vi "FipsAdjacent.vi"() -> (11 "Fips":i32[](array[numeric]))   [LabVIEW 2017] (continued)
MO\"\t29017\t\"Wayne County, MO\"\t29223\n\"Boone County, MO\"\t29019\t\"Audrain County, MO\"\t29007\n\"Boone County, MO\"\t29019\t\"Boone County, MO\"\t29019\n\"Boone County, MO\"\t29019\t\"Callaway County, MO\"\t29027\n\"Boone County, MO\"\t29019\t\"Cole County, MO\"\t29051\n\"Boone County, MO\"\t29019\t\"Cooper County, MO\"\t29053\n\"Boone County, MO\"\t29019\t\"Howard County, MO\"\t29089\n\"Boone County, MO\"\t29019\t\"Moniteau County, MO\"\t29135\n\"Boone County, MO\"\t29019\t\"Randolph County, MO\"\t29175\n\"Buchanan County, MO\"\t29021\t\"Atchison County, KS\"\t20005\n\"Buchanan County, MO\"\t29021\t\"Doniphan County, KS\"\t20043\n\"Buchanan County, MO\"\t29021\t\"Andrew County, MO\"\t29003\n\"Buchanan County, MO\"\t29021\t\"Buchanan County, MO\"\t29021\n\"Buchanan County, MO\"\t29021\t\"Clinton County, MO\"\t29049\n\"Buchanan County, MO\"\t29021\t\"DeKalb County, MO\"\t29063\n\"Buchanan County, MO\"\t29021\t\"Platte County, MO\"\t29165\n\"Butler County, MO\"\t29023\t\"Clay County, AR\"\t05021\n\"Butler County, MO\"\t29023\t\"Butler County, MO\"\t29023\n\"Butler County, MO\"\t29023\t\"Carter County, MO\"\t29035\n\"Butler County, MO\"\t29023\t\"Dunklin County, MO\"\t29069\n\"Butler County, MO\"\t29023\t\"Ripley County, MO\"\t29181\n\"Butler County, MO\"\t29023\t\"Stoddard County, MO\"\t29207\n\"Butler County, MO\"\t29023\t\"Wayne County, MO\"\t29223\n\"Caldwell County, MO\"\t29025\t\"Caldwell County, MO\"\t29025\n\"Caldwell County, MO\"\t29025\t\"Carroll County, MO\"\t29033\n\"Caldwell County, MO\"\t29025\t\"Clinton County, MO\"\t29049\n\"Caldwell County, MO\"\t29025\t\"Daviess County, MO\"\t29061\n\"Caldwell County, MO\"\t29025\t\"DeKalb County, MO\"\t29063\n\"Caldwell County, MO\"\t29025\t\"Livingston County, MO\"\t29117\n\"Caldwell County, MO\"\t29025\t\"Ray County, MO\"\t29177\n\"Callaway County, MO\"\t29027\t\"Audrain County, MO\"\t29007\n\"Callaway County, MO\"\t29027\t\"Boone County, MO\"\t29019\n\"Callaway County, MO\"\t29027\t\"Callaway County, MO\"\t29027\n\"Callaway County, MO\"\t29027\t\"Cole County, MO\"\t29051\n\"Callaway County, MO\"\t29027\t\"Montgomery County, MO\"\t29139\n\"Callaway County, MO\"\t29027\t\"Osage County, MO\"\t29151\n\"Camden County, MO\"\t29029\t\"Benton County, MO\"\t29015\n\"Camden County, MO\"\t29029\t\"Camden County, MO\"\t29029\n\"Camden County, MO\"\t29029\t\"Dallas County, MO\"\t29059\n\"Camden County, MO\"\t29029\t\"Hickory County, MO\"\t29085\n\"Camden County, MO\"\t29029\t\"Laclede County, MO\"\t29105\n\"Camden County, MO\"\t29029\t\"Miller County, MO\"\t29131\n\"Camden County, MO\"\t29029\t\"Morgan County, MO\"\t29141\n\"Camden County, MO\"\t29029\t\"Pulaski County, MO\"\t29169\n\"Cape Girardeau County, MO\"\t29031\t\"Alexander County, IL\"\t17003\n\"Cape Girardeau County, MO\"\t29031\t\"Union County, IL\"\t17181\n\"Cape Girardeau County, MO\"\t29031\t\"Bollinger County, MO\"\t29017\n\"Cape Girardeau County, MO\"\t29031\t\"Cape Girardeau County, MO\"\t29031\n\"Cape Girardeau County, MO\"\t29031\t\"Perry County, MO\"\t29157\n\"Cape Girardeau County, MO\"\t29031\t\"Scott County, MO\"\t29201\n\"Cape Girardeau County, MO\"\t29031\t\"Stoddard County, MO\"\t29207\n\"Carroll County, MO\"\t29033\t\"Caldwell County, MO\"\t29025\n\"Carroll County, MO\"\t29033\t\"Carroll County, MO\"\t29033\n\"Carroll County, MO\"\t29033\t\"Chariton County, MO\"\t29041\n\"Carroll County, MO\"\t29033\t\"Lafayette County, MO\"\t29107\n\"Carroll County, MO\"\t29033\t\"Livingston County, MO\"\t29117\n\"Carroll County, MO\"\t29033\t\"Ray County, MO\"\t29177\n\"Carroll County, MO\"\t29033\t\"Saline County, MO\"\t29195\n\"Carter County, MO\"\t29035\t\"Butler County, MO\"\t29023\n\"Carter County, MO\"\t29035\t\"Carter County, MO\"\t29035\n\"Carter County, MO\"\t29035\t\"Oregon County, MO\"\t29149\n\"Carter County, MO\"\t29035\t\"Reynolds County, MO\"\t29179\n\"Carter County, MO\"\t29035\t\"Ripley County, MO\"\t29181\n\"Carter County, MO\"\t29035\t\"Shannon County, MO\"\t29203\n\"Carter County, MO\"\t29035\t\"Wayne County, MO\"\t29223\n\"Cass County, MO\"\t29037\t\"Johnson County, KS\"\t20091\n\"Cass County, MO\"\t29037\t\"Miami County, KS\"\t20121\n\"Cass County, MO\"\t29037\t\"Bates County, MO\"\t29013\n\"Cass County, MO\"\t29037\t\"Cass County, MO\"\t29037\n\"Cass County, MO\"\t29037\t\"Henry County, MO\"\t29083\n\"Cass County, MO\"\t29037\t\"Jackson County, MO\"\t29095\n\"Cass County, MO\"\t29037\t\"Johnson County, MO\"\t29101\n\"Cedar County, MO\"\t29039\t\"Barton County, MO\"\t29011\n\"Cedar County, MO\"\t29039\t\"Cedar County, MO\"\t29039\n\"Cedar County, MO\"\t29039\t\"Dade County, MO\"\t29057\n\"Cedar County, MO\"\t29039\t\"Polk County, MO\"\t29167\n\"Cedar County, MO\"\t29039\t\"St. Clair County, MO\"\t29185\n\"Cedar County, MO\"\t29039\t\"Vernon County, MO\"\t29217\n\"Chariton County, MO\"\t29041\t\"Carroll County, MO\"\t29033\n\"Chariton County, MO\"\t29041\t\"Chariton County, MO\"\t29041\n\"Chariton County, MO\"\t29041\t\"Howard County, MO\"\t29089\n\"Chariton County, MO\"\t29041\t\"Linn County, MO\"\t29115\n\"Chariton County, MO\"\t29041\t\"Livingston County, MO\"\t29117\n\"Chariton County, MO\"\t29041\t\"Macon County, MO\"\t29121\n\"Chariton County, MO\"\t29041\t\"Randolph County, MO\"\t29175\n\"Chariton County, MO\"\t29041\t\"Saline County, MO\"\t29195\n\"Christian County, MO\"\t29043\t\"Christian County, MO\"\t29043\n\"Christian County, MO\"\t29043\t\"Douglas County, MO\"\t29067\n\"Christian County, MO\"\t29043\t\"Greene County, MO\"\t29077\n\"Christian County, MO\"\t29043\t\"Lawrence County, MO\"\t29109\n\"Christian County, MO\"\t29043\t\"Stone County, MO\"\t29209\n\"Christian County, MO\"\t29043\t\"Taney County, MO\"\t29213\n\"Christian County, MO\"\t29043\t\"Webster County, MO\"\t29225\n\"Clark County, MO\"\t29045\t\"Hancock County, IL\"\t17067\n\"Clark County, MO\"\t29045\t\"Lee County, IA\"\t19111\n\"Clark County, MO\"\t29045\t\"Van Buren County, IA\"\t19177\n\"Clark County, MO\"\t29045\t\"Clark County, MO\"\t29045\n\"Clark County, MO\"\t29045\t\"Knox County, MO\"\t29103\n\"Clark County, MO\"\t29045\t\"Lewis County, MO\"\t29111\n\"Clark County, MO\"\t29045\t\"Scotland County, MO\"\t29199\n\"Clay County, MO\"\t29047\t\"Wyandotte County, KS\"\t20209\n\"Clay County, MO\"\t29047\t\"Clay County, MO\"\t29047\n\"Clay County, MO\"\t29047\t\"Clinton County, MO\"\t29049\n\"Clay County, MO\"\t29047\t\"Jackson County, MO\"\t29095\n\"Clay County, MO\"\t29047\t\"Platte County, MO\"\t29165\n\"Clay County, MO\"\t29047\t\"Ray County, MO\"\t29177\n\"Clinton County, MO\"\t29049\t\"Buchanan County, MO\"\t29021\n\"Clinton County, MO\"\t29049\t\"Caldwell County, MO\"\t29025\n\"Clinton County, MO\"\t29049\t\"Clay County, MO\"\t29047\n\"Clinton County, MO\"\t29049\t\"Clinton County, MO\"\t29049\n\"Clinton County, MO\"\t29049\t\"DeKalb County, MO\"\t29063\n\"Clinton County, MO\"\t29049\t\"Platte County, MO\"\t29165\n\"Clinton County, MO\"\t29049\t\"Ray County, MO\"\t29177\n\"Cole County, MO\"\t29051\t\"Boone County, MO\"\t29019\n\"Cole County, MO\"\t29051\t\"Callaway County, MO\"\t29027\n\"Cole County, MO\"\t29051\t\"Cole County, MO\"\t29051\n\"Cole County, MO\"\t29051\t\"Miller County, MO\"\t29131\n\"Cole County, MO\"\t29051\t\"Moniteau County, MO\"\t29135\n\"Cole County, MO\"\t29051\t\"Osage County, MO\"\t29151\n\"Cooper County, MO\"\t29053\t\"Boone County, MO\"\t29019\n\"Cooper County, MO\"\t29053\t\"Cooper County, MO\"\t29053\n\"Cooper County, MO\"\t29053\t\"Howard County, MO\"\t29089\n\"Cooper County, MO\"\t29053\t\"Moniteau County, MO\"\t29135\n\"Cooper County, MO\"\t29053\t\"Morgan County, MO\"\t29141\n\"Cooper County, MO\"\t29053\t\"Pettis County, MO\"\t29159\n\"Cooper County, MO\"\t29053\t\"Saline County, MO\"\t29195\n\"Crawford County, MO\"\t29055\t\"Crawford County, MO\"\t29055\n\"Crawford County, MO\"\t29055\t\"Dent County, MO\"\t29065\n\"Crawford County, MO\"\t29055\t\"Franklin County, MO\"\t29071\n\"Crawford County, MO\"\t29055\t\"Gasconade County, MO\"\t29073\n\"Crawford County, MO\"\t29055\t\"Iron County, MO\"\t29093\n\"Crawford County, MO\"\t29055\t\"Phelps County, MO\"\t29161\n\"Crawford County, MO\"\t29055\t\"Washington County, MO\"\t29221\n\"Dade County, MO\"\t29057\t\"Barton County, MO\"\t29011\n\"Dade County, MO\"\t29057\t\"Cedar County, MO\"\t29039\n\"Dade County, MO\"\t29057\t\"Dade County, MO\"\t29057\n\"Dade County, MO\"\t29057\t\"Greene County, MO\"\t29077\n\"Dade County, MO\"\t29057\t\"Jasper County, MO\"\t29097\n\"Dade County, MO\"\t29057\t\"Lawrence County, MO\"\t29109\n\"Dade County, MO\"\t29057\t\"Polk County, MO\"\t29167\n\"Dallas County, MO\"\t29059\t\"Camden County, MO\"\t29029\n\"Dallas County, MO\"\t29059\t\"Dallas County, MO\"\t29059\n\"Dallas County, MO\"\t29059\t\"Greene County, MO\"\t29077\n\"Dallas County, MO\"\t29059\t\"Hickory County, MO\"\t29085\n\"Dallas County, MO\"\t29059\t\"Laclede County, MO\"\t29105\n\"Dallas County, MO\"\t29059\t\"Polk County, MO\"\t29167\n\"Dallas County, MO\"\t29059\t\"Webster County, MO\"\t29225\n\"Daviess County, MO\"\t29061\t\"Caldwell County, MO\"\t29025\n\"Daviess County, MO\"\t29061\t\"Daviess County, MO\"\t29061\n\"Daviess County, MO\"\t29061\t\"DeKalb County, MO\"\t29063\n\"Daviess County, MO\"\t29061\t\"Gentry County, MO\"\t29075\n\"Daviess County, MO\"\t29061\t\"Grundy County, MO\"\t29079\n\"Daviess County, MO\"\t29061\t\"Harrison County, MO\"\t29081\n\"Daviess County, MO\"\t29061\t\"Livingston County, MO\"\t29117\n\"DeKalb County, MO\"\t29063\t\"Andrew County, MO\"\t29003\n\"DeKalb County, MO\"\t29063\t\"Buchanan County, MO\"\t29021\n\"DeKalb County, MO\"\t29063\t\"Caldwell County, MO\"\t29025\n\"DeKalb County, MO\"\t29063\t\"Clinton County, MO\"\t29049\n\"DeKalb County, MO\"\t29063\t\"Daviess County, MO\"\t29061\n\"DeKalb County, MO\"\t29063\t\"DeKalb County, MO\"\t29063\n\"DeKalb County, MO\"\t29063\t\"Gentry County, MO\"\t29075\n\"Dent County, MO\"\t29065\t\"Crawford County, MO\"\t29055\n\"Dent County, MO\"\t29065\t\"Dent County, MO\"\t29065\n\"Dent County, MO\"\t29065\t\"Iron County, MO\"\t29093\n\"Dent County, MO\"\t29065\t\"Phelps County, MO\"\t29161\n\"Dent County, MO\"\t29065\t\"Reynolds County, MO\"\t29179\n\"Dent County, MO\"\t29065\t\"Shannon County, MO\"\t29203\n\"Dent County, MO\"\t29065\t\"Texas County, MO\"\t29215\n\"Douglas County, MO\"\t29067\t\"Christian County, MO\"\t29043\n\"Douglas County, MO\"\t29067\t\"Douglas County, MO\"\t29067\n\"Douglas County, MO\"\t29067\t\"Howell County, MO\"\t29091\n\"Douglas County, MO\"\t29067\t\"Ozark County, MO\"\t29153\n\"Douglas County, MO\"\t29067\t\"Taney County, MO\"\t29213\n\"Douglas County, MO\"\t29067\t\"Texas County, MO\"\t29215\n\"Douglas County, MO\"\t29067\t\"Webster County, MO\"\t29225\n\"Douglas County, MO\"\t29067\t\"Wright County, MO\"\t29229\n\"Dunklin County, MO\"\t29069\t\"Clay County, AR\"\t05021\n\"Dunklin County, MO\"\t29069\t\"Craighead County, AR\"\t05031\n\"Dunklin County, MO\"\t29069\t\"Greene County, AR\"\t05055\n\"Dunklin County, MO\"\t29069\t\"Mississippi County, AR\"\t05093\n\"Dunklin County, MO\"\t29069\t\"Butler County, MO\"\t29023\n\"Dunklin County, MO\"\t29069\t\"Dunklin County, MO\"\t29069\n\"Dunklin County, MO\"\t29069\t\"New Madrid County, MO\"\t29143\n\"Dunklin County, MO\"\t29069\t\"Pemiscot County, MO\"\t29155\n\"Dunklin County, MO\"\t29069\t\"Stoddard County, MO\"\t29207\n\"Franklin County, MO\"\t29071\t\"Crawford County, MO\"\t29055\n\"Franklin County, MO\"\t29071\t\"Franklin County, MO\"\t29071\n\"Franklin County, MO\"\t29071\t\"Gasconade County, MO\"\t29073\n\"Franklin County, MO\"\t29071\t\"Jefferson County, MO\"\t29099\n\"Franklin County, MO\"\t29071\t\"St. Charles County, MO\"\t29183\n\"Franklin County, MO\"\t29071\t\"St. Louis County, MO\"\t29189\n\"Franklin County, MO\"\t29071\t\"Warren County, MO\"\t29219\n\"Franklin County, MO\"\t29071\t\"Washington County, MO\"\t29221\n\"Gasconade County, MO\"\t29073\t\"Crawford County, MO\"\t29055\n\"Gasconade County, MO\"\t29073\t\"Franklin County, MO\"\t29071\n\"Gasconade County, MO\"\t29073\t\"Gasconade County, MO\"\t29073\n\"Gasconade County, MO\"\t29073\t\"Maries County, MO\"\t29125\n\"Gasconade County, MO\"\t29073\t\"Montgomery County, MO\"\t29139\n\"Gasconade County, MO\"\t29073\t\"Osage County, MO\"\t29151\n\"Gasconade County, MO\"\t29073\t\"Phelps County, MO\"\t29161\n\"Gasconade County, MO\"\t29073\t\"Warren County, MO\"\t29219\n\"Gentry County, MO\"\t29075\t\"Andrew County, MO\"\t29003\n\"Gentry County, MO\"\t29075\t\"Daviess County, MO\"\t29061\n\"Gentry County, MO\"\t29075\t\"DeKalb County, MO\"\t29063\n\"Gentry County, MO\"\t29075\t\"Gentry County, MO\"\t29075\n\"Gentry County, MO\"\t29075\t\"Harrison County, MO\"\t29081\n\"Gentry County, MO\"\t29075\t\"Nodaway County, MO\"\t29147\n\"Gentry County, MO\"\t29075\t\"Worth County, MO\"\t29227\n\"Greene County, MO\"\t29077\t\"Christian County, MO\"\t29043\n\"Greene County, MO\"\t29077\t\"Dade County, MO\"\t29057\n\"Greene County, MO\"\t29077\t\"Dallas County, MO\"\t29059\n\"Greene County, MO\"\t29077\t\"Greene County, MO\"\t29077\n\"Greene County, MO\"\t29077\t\"Lawrence County, MO\"\t29109\n\"Greene County, MO\"\t29077\t\"Polk County, MO\"\t29167\n\"Greene County, MO\"\t29077\t\"Webster County, MO\"\t29225\n\"Grundy County, MO\"\t29079\t\"Daviess County, MO\"\t29061\n\"Grundy County, MO\"\t29079\t\"Grundy County, MO\"\t29079\n\"Grundy County, MO\"\t29079\t\"Harrison County, MO\"\t29081\n\"Grundy County, MO\"\t29079\t\"Linn County, MO\"\t29115\n\"Grundy County, MO\"\t29079\t\"Livingston County, MO\"\t29117\n\"Grundy County, MO\"\t29079\t\"Mercer County, MO\"\t29129\n\"Grundy County, MO\"\t29079\t\"Sullivan County, MO\"\t29211\n\"Harrison County, MO\"\t29081\t\"Decatur County, IA\"\t19053\n\"Harrison County, MO\"\t29081\t\"Ringgold County, IA\"\t19159\n\"Harrison County, MO\"\t29081\t\"Daviess County, MO\"\t29061\n\"Harrison County, MO\"\t29081\t\"Gentry County, MO\"\t29075\n\"Harrison County, MO\"\t29081\t\"Grundy County, MO\"\t29079\n\"Harrison County, MO\"\t29081\t\"Harrison County, MO\"\t29081\n\"Harrison County, MO\"\t29081\t\"Mercer County, MO\"\t29129\n\"Harrison County, MO\"\t29081\t\"Worth County, MO\"\t29227\n\"Henry County, MO\"\t29083\t\"Bates County, MO\"\t29013\n\"Henry County, MO\"\t29083\t\"Benton County, MO\"\t29015\n\"Henry County, MO\"\t29083\t\"Cass County, MO\"\t29037\n\"Henry County, MO\"\t29083\t\"Henry County, MO\"\t29083\n\"Henry County, MO\"\t29083\t\"Johnson County, MO\"\t29101\n\"Henry County, MO\"\t29083\t\"Pettis County, MO\"\t29159\n\"Henry County, MO\"\t29083\t\"St. Clair County, MO\"\t29185\n\"Hickory County, MO\"\t29085\t\"Benton County, MO\"\t29015\n\"Hickory County, MO\"\t29085\t\"Camden County, MO\"\t29029\n\"Hickory County, MO\"\t29085\t\"Dallas County, MO\"\t29059\n\"Hickory County, MO\"\t29085\t\"Hickory County, MO\"\t29085\n\"Hickory County, MO\"\t29085\t\"Polk County, MO\"\t29167\n\"Hickory County, MO\"\t29085\t\"St. Clair County, MO\"\t29185\n\"Holt County, MO\"\t29087\t\"Doniphan County, KS\"\t20043\n\"Holt County, MO\"\t29087\t\"Andrew County, MO\"\t29003\n\"Holt County, MO\"\t29087\t\"Atchison County, MO\"\t29005\n\"Holt County, MO\"\t29087\t\"Holt County, MO\"\t29087\n\"Holt County, MO\"\t29087\t\"Nodaway County, MO\"\t29147\n\"Holt County, MO\"\t29087\t\"Nemaha County, NE\"\t31127\n\"Holt County, MO\"\t29087\t\"Richardson County, NE\"\t31147\n\"Howard County, MO\"\t29089\t\"Boone County, MO\"\t29019\n\"Howard County, MO\"\t29089\t\"Chariton County, MO\"\t29041\n\"Howard County, MO\"\t29089\t\"Cooper County, MO\"\t29053\n\"Howard County, MO\"\t29089\t\"Howard County, MO\"\t29089\n\"Howard County, MO\"\t29089\t\"Randolph County, MO\"\t29175\n\"Howard County, MO\"\t29089\t\"Saline County, MO\"\t29195\n\"Howell County, MO\"\t29091\t\"Fulton County, AR\"\t05049\n\"Howell County, MO\"\t29091\t\"Douglas County, MO\"\t29067\n\"Howell County, MO\"\t29091\t\"Howell County, MO\"\t29091\n\"Howell County, MO\"\t29091\t\"Oregon County, MO\"\t29149\n\"Howell County, MO\"\t29091\t\"Ozark County, MO\"\t29153\n\"Howell County, MO\"\t29091\t\"Shannon County, MO\"\t29203\n\"Howell County, MO\"\t29091\t\"Texas County, MO\"\t29215\n\"Iron County, MO\"\t29093\t\"Crawford County, MO\"\t29055\n\"Iron County, MO\"\t29093\t\"Dent County, MO\"\t29065\n\"Iron County, MO\"\t29093\t\"Iron County, MO\"\t29093\n\"Iron County, MO\"\t29093\t\"Madison County, MO\"\t29123\n\"Iron County, MO\"\t29093\t\"Reynolds County, MO\"\t29179\n\"Iron County, MO\"\t29093\t\"St. Francois County, MO\"\t29187\n\"Iron County, MO\"\t29093\t\"Washington County, MO\"\t29221\n\"Iron County, MO\"\t29093\t\"Wayne County, MO\"\t29223\n\"Jackson County, MO\"\t29095\t\"Johnson County, KS\"\t20091\n\"Jackson County, MO\"\t29095\t\"Wyandotte County, KS\"\t20209\n\"Jackson County, MO\"\t29095\t\"Cass County, MO\"\t29037\n\"Jackson County, MO\"\t29095\t\"Clay County, MO\"\t29047\n\"Jackson County, MO\"\t29095\t\"Jackson County, MO\"\t29095\n\"Jackson County, MO\"\t29095\t\"Johnson County, MO\"\t29101\n\"Jackson County, MO\"\t29095\t\"Lafayette County, MO\"\t29107\n\"Jackson County, MO\"\t29095\t\"Ray County, MO\"\t29177\n\"Jasper County, MO\"\t29097\t\"Cherokee County, KS\"\t20021\n\"Jasper County, MO\"\t29097\t\"Crawford County, KS\"\t20037\n\"Jasper County, MO\"\t29097\t\"Barton County, MO\"\t29011\n\"Jasper County, MO\"\t29097\t\"Dade County, MO\"\t29057\n\"Jasper County, MO\"\t29097\t\"Jasper County, MO\"\t29097\n\"Jasper County, MO\"\t29097\t\"Lawrence County, MO\"\t29109\n\"Jasper County, MO\"\t29097\t\"Newton County, MO\"\t29145\n\"Jefferson County, MO\"\t29099\t\"Monroe County, IL\"\t17133\n\"Jefferson County, MO\"\t29099\t\"Franklin County, MO\"\t29071\n\"Jefferson County, MO\"\t29099\t\"Jefferson County, MO\"\t29099\n\"Jefferson County, MO\"\t29099\t\"Ste. Genevieve County, MO\"\t29186\n\"Jefferson County, MO\"\t29099\t\"St. Francois County, MO\"\t29187\n\"Jefferson County, MO\"\t29099\t\"St. Louis County, MO\"\t29189\n\"Jefferson County, MO\"\t29099\t\"Washington County, MO\"\t29221\n\"Johnson County, MO\"\t29101\t\"Cass County, MO\"\t29037\n\"Johnson County, MO\"\t29101\t\"Henry County, MO\"\t29083\n\"Johnson County, MO\"\t29101\t\"Jackson County, MO\"\t29095\n\"Johnson County, MO\"\t29101\t\"Johnson County, MO\"\t29101\n\"Johnson County, MO\"\t29101\t\"Lafayette County, MO\"\t29107\n\"Johnson County, MO\"\t29101\t\"Pettis County, MO\"\t29159\n\"Knox County, MO\"\t29103\t\"Adair County, MO\"\t29001\n\"Knox County, MO\"\t29103\t\"Clark County, MO\"\t29045\n\"Knox County, MO\"\t29103\t\"Knox County, MO\"\t29103\n\"Knox County, MO\"\t29103\t\"Lewis County, MO\"\t29111\n\"Knox County, MO\"\t29103\t\"Macon County, MO\"\t29121\n\"Knox County, MO\"\t29103\t\"Scotland County, MO\"\t29199\n\"Knox County, MO\"\t29103\t\"Shelby County, MO\"\t29205\n\"Laclede County, MO\"\t29105\t\"Camden County, MO\"\t29029\n\"Laclede County, MO\"\t29105\t\"Dallas County, MO\"\t29059\n\"Laclede County, MO\"\t29105\t\"Laclede County, MO\"\t29105\n\"Laclede County, MO\"\t29105\t\"Pulaski County, MO\"\t29169\n\"Laclede County, MO\"\t29105\t\"Texas County, MO\"\t29215\n\"Laclede County, MO\"\t29105\t\"Webster County, MO\"\t29225\n\"Laclede County, MO\"\t29105\t\"Wright County, MO\"\t29229\n\"Lafayette County, MO\"\t29107\t\"Carroll County, MO\"\t29033\n\"Lafayette County, MO\"\t29107\t\"Jackson County, MO\"\t29095\n\"Lafayette County, MO\"\t29107\t\"Johnson County, MO\"\t29101\n\"Lafayette County, MO\"\t29107\t\"Lafayette County, MO\"\t29107\n\"Lafayette County, MO\"\t29107\t\"Pettis County, MO\"\t29159\n\"Lafayette County, MO\"\t29107\t\"Ray County, MO\"\t29177\n\"Lafayette County, MO\"\t29107\t\"Saline County, MO\"\t29195\n\"Lawrence County, MO\"\t29109\t\"Barry County, MO\"\t29009\n\"Lawrence County, MO\"\t29109\t\"Christian County, MO\"\t29043\n\"Lawrence County, MO\"\t29109\t\"Dade County, MO\"\t29057\n\"Lawrence County, MO\"\t29109\t\"Greene County, MO\"\t29077\n\"Lawrence County, MO\"\t29109\t\"Jasper County, MO\"\t29097\n\"Lawrence County, MO\"\t29109\t\"Lawrence County, MO\"\t29109\n\"Lawrence County, MO\"\t29109\t\"Newton County, MO\"\t29145\n\"Lawrence County, MO\"\t29109\t\"Stone County, MO\"\t29209\n\"Lewis County, MO\"\t29111\t\"Adams County, IL\"\t17001\n\"Lewis County, MO\"\t29111\t\"Hancock County, IL\"\t17067\n\"Lewis County, MO\"\t29111\t\"Clark County, MO\"\t29045\n\"Lewis County, MO\"\t29111\t\"Knox County, MO\"\t29103\n\"Lewis County, MO\"\t29111\t\"Lewis County, MO\"\t29111\n\"Lewis County, MO\"\t29111\t\"Marion County, MO\"\t29127\n\"Lewis County, MO\"\t29111\t\"Shelby County, MO\"\t29205\n\"Lincoln County, MO\"\t29113\t\"Calhoun County, IL\"\t17013\n\"Lincoln County, MO\"\t29113\t\"Lincoln County, MO\"\t29113\n\"Lincoln County, MO\"\t29113\t\"Montgomery County, MO\"\t29139\n\"Lincoln County, MO\"\t29113\t\"Pike County, MO\"\t29163\n\"Lincoln County, MO\"\t29113\t\"St. Charles County, MO\"\t29183\n\"Lincoln County, MO\"\t29113\t\"Warren County, MO\"\t29219\n\"Linn County, MO\"\t29115\t\"Adair County, MO\"\t29001\n\"Linn County, MO\"\t29115\t\"Chariton County, MO\"\t29041\n\"Linn County, MO\"\t29115\t\"Grundy County, MO\"\t29079\n\"Linn County, MO\"\t29115\t\"Linn County, MO\"\t29115\n\"Linn County, MO\"\t29115\t\"Livingston County, MO\"\t29117\n\"Linn County, MO\"\t29115\t\"Macon County, MO\"\t29121\n\"Linn County, MO\"\t29115\t\"Sullivan County, MO\"\t29211\n\"Livingston County, MO\"\t29117\t\"Caldwell County, MO\"\t29025\n\"Livingston County, MO\"\t29117\t\"Carroll County, MO\"\t29033\n\"Livingston County, MO\"\t29117\t\"Chariton County, MO\"\t29041\n\"Livingston County, MO\"\t29117\t\"Daviess County, MO\"\t29061\n\"Livingston County, MO\"\t29117\t\"Grundy County, MO\"\t29079\n\"Livingston County, MO\"\t29117\t\"Linn County, MO\"\t29115\n\"Livingston County, MO\"\t29117\t\"Livingston County, MO\"\t29117\n\"McDonald County, MO\"\t29119\t\"Benton County, AR\"\t05007\n\"McDonald County, MO\"\t29119\t\"Barry County, MO\"\t29009\n\"McDonald County, MO\"\t29119\t\"McDonald County, MO\"\t29119\n\"McDonald County, MO\"\t29119\t\"Newton County, MO\"\t29145\n\"McDonald County, MO\"\t29119\t\"Delaware County, OK\"\t40041\n\"McDonald County, MO\"\t29119\t\"Ottawa County, OK\"\t40115\n\"Macon County, MO\"\t29121\t\"Adair County, MO\"\t29001\n\"Macon County, MO\"\t29121\t\"Chariton County, MO\"\t29041\n\"Macon County, MO\"\t29121\t\"Knox County, MO\"\t29103\n\"Macon County, MO\"\t29121\t\"Linn County, MO\"\t29115\n\"Macon County, MO\"\t29121\t\"Macon County, MO\"\t29121\n\"Macon County, MO\"\t29121\t\"Monroe County, MO\"\t29137\n\"Macon County, MO\"\t29121\t\"Randolph County, MO\"\t29175\n\"Macon County, MO\"\t29121\t\"Shelby County, MO\"\t29205\n\"Madison County, MO\"\t29123\t\"Bollinger County, MO\"\t29017\n\"Madison County, MO\"\t29123\t\"Iron County, MO\"\t29093\n\"Madison County, MO\"\t29123\t\"Madison County, MO\"\t29123\n\"Madison County, MO\"\t29123\t\"Perry County, MO\"\t29157\n\"Madison County, MO\"\t29123\t\"St. Francois County, MO\"\t29187\n\"Madison County, MO\"\t29123\t\"Wayne County, MO\"\t29223\n\"Maries County, MO\"\t29125\t\"Gasconade County, MO\"\t29073\n\"Maries County, MO\"\t29125\t\"Maries County, MO\"\t29125\n\"Maries County, MO\"\t29125\t\"Miller County, MO\"\t29131\n\"Maries County, MO\"\t29125\t\"Osage County, MO\"\t29151\n\"Maries County, MO\"\t29125\t\"Phelps County, MO\"\t29161\n\"Maries County, MO\"\t29125\t\"Pulaski County, MO\"\t29169\n\"Marion County, MO\"\t29127\t\"Adams County, IL\"\t17001\n\"Marion County, MO\"\t29127\t\"Pike County, IL\"\t17149\n\"Marion County, MO\"\t29127\t\"Lewis County, MO\"\t29111\n\"Marion County, MO\"\t29127\t\"Marion County, MO\"\t29127\n\"Marion County, MO\"\t29127\t\"Monroe County, MO\"\t29137\n\"Marion County, MO\"\t29127\t\"Ralls County, MO\"\t29173\n\"Marion County, MO\"\t29127\t\"Shelby County, MO\"\t29205\n\"Mercer County, MO\"\t29129\t\"Decatur County, IA\"\t19053\n\"Mercer County, MO\"\t29129\t\"Wayne County, IA\"\t19185\n\"Mercer County, MO\"\t29129\t\"Grundy County, MO\"\t29079\n\"Mercer County, MO\"\t29129\t\"Harrison County, MO\"\t29081\n\"Mercer County, MO\"\t29129\t\"Mercer County, MO\"\t29129\n\"Mercer County, MO\"\t29129\t\"Putnam County, MO\"\t29171\n\"Mercer County, MO\"\t29129\t\"Sullivan County, MO\"\t29211\n\"Miller County, MO\"\t29131\t\"Camden County, MO\"\t29029\n\"Miller County, MO\"\t29131\t\"Cole County, MO\"\t29051\n\"Miller County, MO\"\t29131\t\"Maries County, MO\"\t29125\n\"Miller County, MO\"\t29131\t\"Miller County, MO\"\t29131\n\"Miller County, MO\"\t29131\t\"Moniteau County, MO\"\t29135\n\"Miller County, MO\"\t29131\t\"Morgan County, MO\"\t29141\n\"Miller County, MO\"\t29131\t\"Osage County, MO\"\t29151\n\"Miller County, MO\"\t29131\t\"Pulaski County, MO\"\t29169\n\"Mississippi County, MO\"\t29133\t\"Alexander County, IL\"\t17003\n\"Mississippi County, MO\"\t29133\t\"Ballard County, KY\"\t21007\n\"Mississippi County, MO\"\t29133\t\"Carlisle County, KY\"\t21039\n\"Mississippi County, MO\"\t29133\t\"Fulton County, KY\"\t21075\n\"Mississippi County, MO\"\t29133\t\"Hickman County, KY\"\t21105\n\"Mississippi County, MO\"\t29133\t\"Mississippi County, MO\"\t29133\n\"Mississippi County, MO\"\t29133\t\"New Madrid County, MO\"\t29143\n\"Mississippi County, MO\"\t29133\t\"Scott County, MO\"\t29201\n\"Moniteau County, MO\"\t29135\t\"Boone County, MO\"\t29019\n\"Moniteau County, MO\"\t29135\t\"Cole County, MO\"\t29051\n\"Moniteau County, MO\"\t29135\t\"Cooper County, MO\"\t29053\n\"Moniteau County, MO\"\t29135\t\"Miller County, MO\"\t29131\n\"Moniteau County, MO\"\t29135\t\"Moniteau County, MO\"\t29135\n\"Moniteau County, MO\"\t29135\t\"Morgan County, MO\"\t29141\n\"Monroe County, MO\"\t29137\t\"Audrain County, MO\"\t29007\n\"Monroe County, MO\"\t29137\t\"Macon County, MO\"\t29121\n\"Monroe County, MO\"\t29137\t\"Marion County, MO\"\t29127\n\"Monroe County, MO\"\t29137\t\"Monroe County, MO\"\t29137\n\"Monroe County, MO\"\t29137\t\"Ralls County, MO\"\t29173\n\"Monroe County, MO\"\t29137\t\"Randolph County, MO\"\t29175\n\"Monroe County, MO\"\t29137\t\"Shelby County, MO\"\t29205\n\"Montgomery County, MO\"\t29139\t\"Audrain County, MO\"\t29007\n\"Montgomery County, MO\"\t29139\t\"Callaway County, MO\"\t29027\n\"Montgomery County, MO\"\t29139\t\"Gasconade County, MO\"\t29073\n\"Montgomery County, MO\"\t29139\t\"Lincoln County, MO\"\t29113\n\"Montgomery County, MO\"\t29139\t\"Montgomery County, MO\"\t29139\n\"Montgomery County, MO\"\t29139\t\"Osage County, MO\"\t29151\n\"Montgomery County, MO\"\t29139\t\"Pike County, MO\"\t29163\n\"Montgomery County, MO\"\t29139\t\"Warren County, MO\"\t29219\n\"Morgan County, MO\"\t29141\t\"Benton County, MO\"\t29015\n\"Morgan County, MO\"\t29141\t\"Camden County, MO\"\t29029\n\"Morgan County, MO\"\t29141\t\"Cooper County, MO\"\t29053\n\"Morgan County, MO\"\t29141\t\"Miller County, MO\"\t29131\n\"Morgan County, MO\"\t29141\t\"Moniteau County, MO\"\t29135\n\"Morgan County, MO\"\t29141\t\"Morgan County, MO\"\t29141\n\"Morgan County, MO\"\t29141\t\"Pettis County, MO\"\t29159\n\"New Madrid County, MO\"\t29143\t\"Fulton County, KY\"\t21075\n\"New Madrid County, MO\"\t29143\t\"Dunklin County, MO\"\t29069\n\"New Madrid County, MO\"\t29143\t\"Mississippi County, MO\"\t29133\n\"New Madrid County, MO\"\t29143\t\"New Madrid County, MO\"\t29143\n\"New Madrid County, MO\"\t29143\t\"Pemiscot County, MO\"\t29155\n\"New Madrid County, MO\"\t29143\t\"Scott County, MO\"\t29201\n\"New Madrid County, MO\"\t29143\t\"Stoddard County, MO\"\t29207\n\"New Madrid County, MO\"\t29143\t\"Lake County, TN\"\t47095\n\"Newton County, MO\"\t29145\t\"Cherokee County, KS\"\t20021\n\"Newton County, MO\"\t29145\t\"Barry County, MO\"\t29009\n\"Newton County, MO\"\t29145\t\"Jasper County, MO\"\t29097\n\"Newton County, MO\"\t29145\t\"Lawrence County, MO\"\t29109\n\"Newton County, MO\"\t29145\t\"McDonald County, MO\"\t29119\n\"Newton County, MO\"\t29145\t\"Newton County, MO\"\t29145\n\"Newton County, MO\"\t29145\t\"Ottawa County, OK\"\t40115\n\"Nodaway County, MO\"\t29147\t\"Page County, IA\"\t19145\n\"Nodaway County, MO\"\t29147\t\"Taylor County, IA\"\t19173\n\"Nodaway County, MO\"\t29147\t\"Andrew County, MO\"\t29003\n\"Nodaway County, MO\"\t29147\t\"Atchison County, MO\"\t29005\n\"Nodaway County, MO\"\t29147\t\"Gentry County, MO\"\t29075\n\"Nodaway County, MO\"\t29147\t\"Holt County, MO\"\t29087\n\"Nodaway County, MO\"\t29147\t\"Nodaway County, MO\"\t29147\n\"Nodaway County, MO\"\t29147\t\"Worth County, MO\"\t29227\n\"Oregon County, MO\"\t29149\t\"Fulton County, AR\"\t05049\n\"Oregon County, MO\"\t29149\t\"Randolph County, AR\"\t05121\n\"Oregon County, MO\"\t29149\t\"Sharp County, AR\"\t05135\n\"Oregon County, MO\"\t29149\t\"Carter County, MO\"\t29035\n\"Oregon County, MO\"\t29149\t\"Howell County, MO\"\t29091\n\"Oregon County, MO\"\t29149\t\"Oregon County, MO\"\t29149\n\"Oregon County, MO\"\t29149\t\"Ripley County, MO\"\t29181\n\"Oregon County, MO\"\t29149\t\"Shannon County, MO\"\t29203\n\"Osage County, MO\"\t29151\t\"Callaway County, MO\"\t29027\n\"Osage County, MO\"\t29151\t\"Cole County, MO\"\t29051\n\"Osage County, MO\"\t29151\t\"Gasconade County, MO\"\t29073\n\"Osage County, MO\"\t29151\t\"Maries County, MO\"\t29125\n\"Osage County, MO\"\t29151\t\"Miller County, MO\"\t29131\n\"Osage County, MO\"\t29151\t\"Montgomery County, MO\"\t29139\n\"Osage County, MO\"\t29151\t\"Osage County, MO\"\t29151\n\"Ozark County, MO\"\t29153\t\"Baxter County, AR\"\t05005\n\"Ozark County, MO\"\t29153\t\"Fulton County, AR\"\t05049\n\"Ozark County, MO\"\t29153\t\"Marion County, AR\"\t05089\n\"Ozark County, MO\"\t29153\t\"Douglas County, MO\"\t29067\n\"Ozark County, MO\"\t29153\t\"Howell County, MO\"\t29091\n\"Ozark County, MO\"\t29153\t\"Ozark County, MO\"\t29153\n\"Ozark County, MO\"\t29153\t\"Taney County, MO\"\t29213\n\"Pemiscot County, MO\"\t29155\t\"Mississippi County, AR\"\t05093\n\"Pemiscot County, MO\"\t29155\t\"Dunklin County, MO\"\t29069\n\"Pemiscot County, MO\"\t29155\t\"New Madrid County, MO\"\t29143\n\"Pemiscot County, MO\"\t29155\t\"Pemiscot County, MO\"\t29155\n\"Pemiscot County, MO\"\t29155\t\"Dyer County, TN\"\t47045\n\"Pemiscot County, MO\"\t29155\t\"Lake County, TN\"\t47095\n\"Perry County, MO\"\t29157\t\"Jackson County, IL\"\t17077\n\"Perry County, MO\"\t29157\t\"Randolph County, IL\"\t17157\n\"Perry County, MO\"\t29157\t\"Union County, IL\"\t17181\n\"Perry County, MO\"\t29157\t\"Bollinger County, MO\"\t29017\n\"Perry County, MO\"\t29157\t\"Cape Girardeau County, MO\"\t29031\n\"Perry County, MO\"\t29157\t\"Madison County, MO\"\t29123\n\"Perry County, MO\"\t29157\t\"Perry County, MO\"\t29157\n\"Perry County, MO\"\t29157\t\"Ste. Genevieve County, MO\"\t29186\n\"Perry County, MO\"\t29157\t\"St. Francois County, MO\"\t29187\n\"Pettis County, MO\"\t29159\t\"Benton County, MO\"\t29015\n\"Pettis County, MO\"\t29159\t\"Cooper County, MO\"\t29053\n\"Pettis County, MO\"\t29159\t\"Henry County, MO\"\t29083\n\"Pettis County, MO\"\t29159\t\"Johnson County, MO\"\t29101\n\"Pettis County, MO\"\t29159\t\"Lafayette County, MO\"\t29107\n\"Pettis County, MO\"\t29159\t\"Morgan County, MO\"\t29141\n\"Pettis County, MO\"\t29159\t\"Pettis County, MO\"\t29159\n\"Pettis County, MO\"\t29159\t\"Saline County, MO\"\t29195\n\"Phelps County, MO\"\t29161\t\"Crawford County, MO\"\t29055\n\"Phelps County, MO\"\t29161\t\"Dent County, MO\"\t29065\n\"Phelps County, MO\"\t29161\t\"Gasconade County, MO\"\t29073\n\"Phelps County, MO\"\t29161\t\"Maries County, MO\"\t29125\n\"Phelps County, MO\"\t29161\t\"Phelps County, MO\"\t29161\n\"Phelps County, MO\"\t29161\t\"Pulaski County, MO\"\t29169\n\"Phelps County, MO\"\t29161\t\"Texas County, MO\"\t29215\n\"Pike County, MO\"\t29163\t\"Calhoun County, IL\"\t17013\n\"Pike County, MO\"\t29163\t\"Pike County, IL\"\t17149\n\"Pike County, MO\"\t29163\t\"Audrain County, MO\"\t29007\n\"Pike County, MO\"\t29163\t\"Lincoln County, MO\"\t29113\n\"Pike County, MO\"\t29163\t\"Montgomery County, MO\"\t29139\n\"Pike County, MO\"\t29163\t\"Pike County, MO\"\t29163\n\"Pike County, MO\"\t29163\t\"Ralls County, MO\"\t29173\n\"Platte County, MO\"\t29165\t\"Atchison County, KS\"\t20005\n\"Platte County, MO\"\t29165\t\"Leavenworth County, KS\"\t20103\n\"Platte County, MO\"\t29165\t\"Wyandotte County, KS\"\t20209\n\"Platte County, MO\"\t29165\t\"Buchanan County, MO\"\t29021\n\"Platte County, MO\"\t29165\t\"Clay County, MO\"\t29047\n\"Platte County, MO\"\t29165\t\"Clinton County, MO\"\t29049\n\"Platte County, MO\"\t29165\t\"Platte County, MO\"\t29165\n\"Polk County, MO\"\t29167\t\"Cedar County, MO\"\t29039\n\"Polk County, MO\"\t29167\t\"Dade County, MO\"\t29057\n\"Polk County, MO\"\t29167\t\"Dallas County, MO\"\t29059\n\"Polk County, MO\"\t29167\t\"Greene County, MO\"\t29077\n\"Polk County, MO\"\t29167\t\"Hickory County, MO\"\t29085\n\"Polk County, MO\"\t29167\t\"Polk County, MO\"\t29167\n\"Polk County, MO\"\t29167\t\"St. Clair County, MO\"\t29185\n\"Pulaski County, MO\"\t29169\t\"Camden County, MO\"\t29029\n\"Pulaski County, MO\"\t29169\t\"Laclede County, MO\"\t29105\n\"Pulaski County, MO\"\t29169\t\"Maries County, MO\"\t29125\n\"Pulaski County, MO\"\t29169\t\"Miller County, MO\"\t29131\n\"Pulaski County, MO\"\t29169\t\"Phelps County, MO\"\t29161\n\"Pulaski County, MO\"\t29169\t\"Pulaski County, MO\"\t29169\n\"Pulaski County, MO\"\t29169\t\"Texas County, MO\"\t29215\n\"Putnam County, MO\"\t29171\t\"Appanoose County, IA\"\t19007\n\"Putnam County, MO\"\t29171\t\"Wayne County, IA\"\t19185\n\"Putnam County, MO\"\t29171\t\"Adair County, MO\"\t29001\n\"Putnam County, MO\"\t29171\t\"Mercer County, MO\"\t29129\n\"Putnam County, MO\"\t29171\t\"Putnam County, MO\"\t29171\n\"Putnam County, MO\"\t29171\t\"Schuyler County, MO\"\t29197\n\"Putnam County, MO\"\t29171\t\"Sullivan County, MO\"\t29211\n\"Ralls County, MO\"\t29173\t\"Pike County, IL\"\t17149\n\"Ralls County, MO\"\t29173\t\"Audrain County, MO\"\t29007\n\"Ralls County, MO\"\t29173\t\"Marion County, MO\"\t29127\n\"Ralls County, MO\"\t29173\t\"Monroe County, MO\"\t29137\n\"Ralls County, MO\"\t29173\t\"Pike County, MO\"\t29163\n\"Ralls County, MO\"\t29173\t\"Ralls County, MO\"\t29173\n\"Randolph County, MO\"\t29175\t\"Audrain County, MO\"\t29007\n\"Randolph County, MO\"\t29175\t\"Boone County, MO\"\t29019\n\"Randolph County, MO\"\t29175\t\"Chariton County, MO\"\t29041\n\"Randolph County, MO\"\t29175\t\"Howard County, MO\"\t29089\n\"Randolph County, MO\"\t29175\t\"Macon County, MO\"\t29121\n\"Randolph County, MO\"\t29175\t\"Monroe County, MO\"\t29137\n\"Randolph County, MO\"\t29175\t\"Randolph County, MO\"\t29175\n\"Ray County, MO\"\t29177\t\"Caldwell County, MO\"\t29025\n\"Ray County, MO\"\t29177\t\"Carroll County, MO\"\t29033\n\"Ray County, MO\"\t29177\t\"Clay County, MO\"\t29047\n\"Ray County, MO\"\t29177\t\"Clinton County, MO\"\t29049\n\"Ray County, MO\"\t29177\t\"Jackson County, MO\"\t29095\n\"Ray County, MO\"\t29177\t\"Lafayette County, MO\"\t29107\n\"Ray County, MO\"\t29177\t\"Ray County, MO\"\t29177\n\"Reynolds County, MO\"\t29179\t\"Carter County, MO\"\t29035\n\"Reynolds County, MO\"\t29179\t\"Dent County, MO\"\t29065\n\"Reynolds County, MO\"\t29179\t\"Iron County, MO\"\t29093\n\"Reynolds County, MO\"\t29179\t\"Reynolds County, MO\"\t29179\n\"Reynolds County, MO\"\t29179\t\"Shannon County, MO\"\t29203\n\"Reynolds County, MO\"\t29179\t\"Wayne County, MO\"\t29223\n\"Ripley County, MO\"\t29181\t\"Clay County, AR\"\t05021\n\"Ripley County, MO\"\t29181\t\"Randolph County, AR\"\t05121\n\"Ripley County, MO\"\t29181\t\"Butler County, MO\"\t29023\n\"Ripley County, MO\"\t29181\t\"Carter County, MO\"\t29035\n\"Ripley County, MO\"\t29181\t\"Oregon County, MO\"\t29149\n\"Ripley County, MO\"\t29181\t\"Ripley County, MO\"\t29181\n\"St. Charles County, MO\"\t29183\t\"Calhoun County, IL\"\t17013\n\"St. Charles County, MO\"\t29183\t\"Jersey County, IL\"\t17083\n\"St. Charles County, MO\"\t29183\t\"Madison County, IL\"\t17119\n\"St. Charles County, MO\"\t29183\t\"Franklin County, MO\"\t29071\n\"St. Charles County, MO\"\t29183\t\"Lincoln County, MO\"\t29113\n\"St. Charles County, MO\"\t29183\t\"St. Charles County, MO\"\t29183\n\"St. Charles County, MO\"\t29183\t\"St. Louis County, MO\"\t29189\n\"St. Charles County, MO\"\t29183\t\"Warren County, MO\"\t29219\n\"St. Clair County, MO\"\t29185\t\"Bates County, MO\"\t29013\n\"St. Clair County, MO\"\t29185\t\"Benton County, MO\"\t29015\n\"St. Clair County, MO\"\t29185\t\"Cedar County, MO\"\t29039\n\"St. Clair County, MO\"\t29185\t\"Henry County, MO\"\t29083\n\"St. Clair County, MO\"\t29185\t\"Hickory County, MO\"\t29085\n\"St. Clair County, MO\"\t29185\t\"Polk County, MO\"\t29167\n\"St. Clair County, MO\"\t29185\t\"St. Clair County, MO\"\t29185\n\"St. Clair County, MO\"\t29185\t\"Vernon County, MO\"\t29217\n\"Ste. Genevieve County, MO\"\t29186\t\"Monroe County, IL\"\t17133\n\"Ste. Genevieve County, MO\"\t29186\t\"Randolph County, IL\"\t17157\n\"Ste. Genevieve County, MO\"\t29186\t\"Jefferson County, MO\"\t29099\n\"Ste. Genevieve County, MO\"\t29186\t\"Perry County, MO\"\t29157\n\"Ste. Genevieve County, MO\"\t29186\t\"Ste. Genevieve County, MO\"\t29186\n\"Ste. Genevieve County, MO\"\t29186\t\"St. Francois County, MO\"\t29187\n\"St. Francois County, MO\"\t29187\t\"Iron County, MO\"\t29093\n\"St. Francois County, MO\"\t29187\t\"Jefferson County, MO\"\t29099\n\"St. Francois County, MO\"\t29187\t\"Madison County, MO\"\t29123\n\"St. Francois County, MO\"\t29187\t\"Perry County, MO\"\t29157\n\"St. Francois County, MO\"\t29187\t\"Ste. Genevieve County, MO\"\t29186\n\"St. Francois County, MO\"\t29187\t\"St. Francois County, MO\"\t29187\n\"St. Francois County, MO\"\t29187\t\"Washington County, MO\"\t29221\n\"St. Louis County, MO\"\t29189\t\"Madison County, IL\"\t17119\n\"St. Louis County, MO\"\t29189\t\"Monroe County, IL\"\t17133\n\"St. Louis County, MO\"\t29189\t\"St. Clair County, IL\"\t17163\n\"St. Louis County, MO\"\t29189\t\"Franklin County, MO\"\t29071\n\"St. Louis County, MO\"\t29189\t\"Jefferson County, MO\"\t29099\n\"St. Louis County, MO\"\t29189\t\"St. Charles County, MO\"\t29183\n\"St. Louis County, MO\"\t29189\t\"St. Louis County, MO\"\t29189\n\"St. Louis County, MO\"\t29189\t\"St. Louis city, MO\"\t29510\n\"Saline County, MO\"\t29195\t\"Carroll County, MO\"\t29033\n\"Saline County, MO\"\t29195\t\"Chariton County, MO\"\t29041\n\"Saline County, MO\"\t29195\t\"Cooper County, MO\"\t29053\n\"Saline County, MO\"\t29195\t\"Howard County, MO\"\t29089\n\"Saline County, MO\"\t29195\t\"Lafayette County, MO\"\t29107\n\"Saline County, MO\"\t29195\t\"Pettis County, MO\"\t29159\n\"Saline County, MO\"\t29195\t\"Saline County, MO\"\t29195\n\"Schuyler County, MO\"\t29197\t\"Appanoose County, IA\"\t19007\n\"Schuyler County, MO\"\t29197\t\"Davis County, IA\"\t19051\n\"Schuyler County, MO\"\t29197\t\"Adair County, MO\"\t29001\n\"Schuyler County, MO\"\t29197\t\"Putnam County, MO\"\t29171\n\"Schuyler County, MO\"\t29197\t\"Schuyler County, MO\"\t29197\n\"Schuyler County, MO\"\t29197\t\"Scotland County, MO\"\t29199\n\"Scotland County, MO\"\t29199\t\"Davis County, IA\"\t19051\n\"Scotland County, MO\"\t29199\t\"Van Buren County, IA\"\t19177\n\"Scotland County, MO\"\t29199\t\"Adair County, MO\"\t29001\n\"Scotland County, MO\"\t29199\t\"Clark County, MO\"\t29045\n\"Scotland County, MO\"\t29199\t\"Knox County, MO\"\t29103\n\"Scotland County, MO\"\t29199\t\"Schuyler County, MO\"\t29197\n\"Scotland County, MO\"\t29199\t\"Scotland County, MO\"\t29199\n\"Scott County, MO\"\t29201\t\"Alexander County, IL\"\t17003\n\"Scott County, MO\"\t29201\t\"Cape Girardeau County, MO\"\t29031\n\"Scott County, MO\"\t29201\t\"Mississippi County, MO\"\t29133\n\"Scott County, MO\"\t29201\t\"New Madrid County, MO\"\t29143\n\"Scott County, MO\"\t29201\t\"Scott County, MO\"\t29201\n\"Scott County, MO\"\t29201\t\"Stoddard County, MO\"\t29207\n\"Shannon County, MO\"\t29203\t\"Carter County, MO\"\t29035\n\"Shannon County, MO\"\t29203\t\"Dent County, MO\"\t29065\n\"Shannon County, MO\"\t29203\t\"Howell County, MO\"\t29091\n\"Shannon County, MO\"\t29203\t\"Oregon County, MO\"\t29149\n\"Shannon County, MO\"\t29203\t\"Reynolds County, MO\"\t29179\n\"Shannon County, MO\"\t29203\t\"Shannon County, MO\"\t29203\n\"Shannon County, MO\"\t29203\t\"Texas County, MO\"\t29215\n\"Shelby County, 
